vi "Get Hardware ID.vi"() -> ()   [LabVIEW 2012]
panel:
  out "stop":bool
  out "Action":string
  out "p 8":bool
  out "p 7":bool
  out "p 6":bool
  out "p 5":bool
  out "p 4":bool
  out "p 3":bool
  out "p 2":bool
  out "p 1":bool
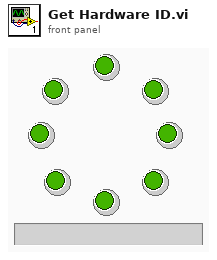
[diagram p1: front panel]
types:
  T1 = enum16{"open", "replace", "create", "open or create", "replace or create", "replace or create with confirmation"}
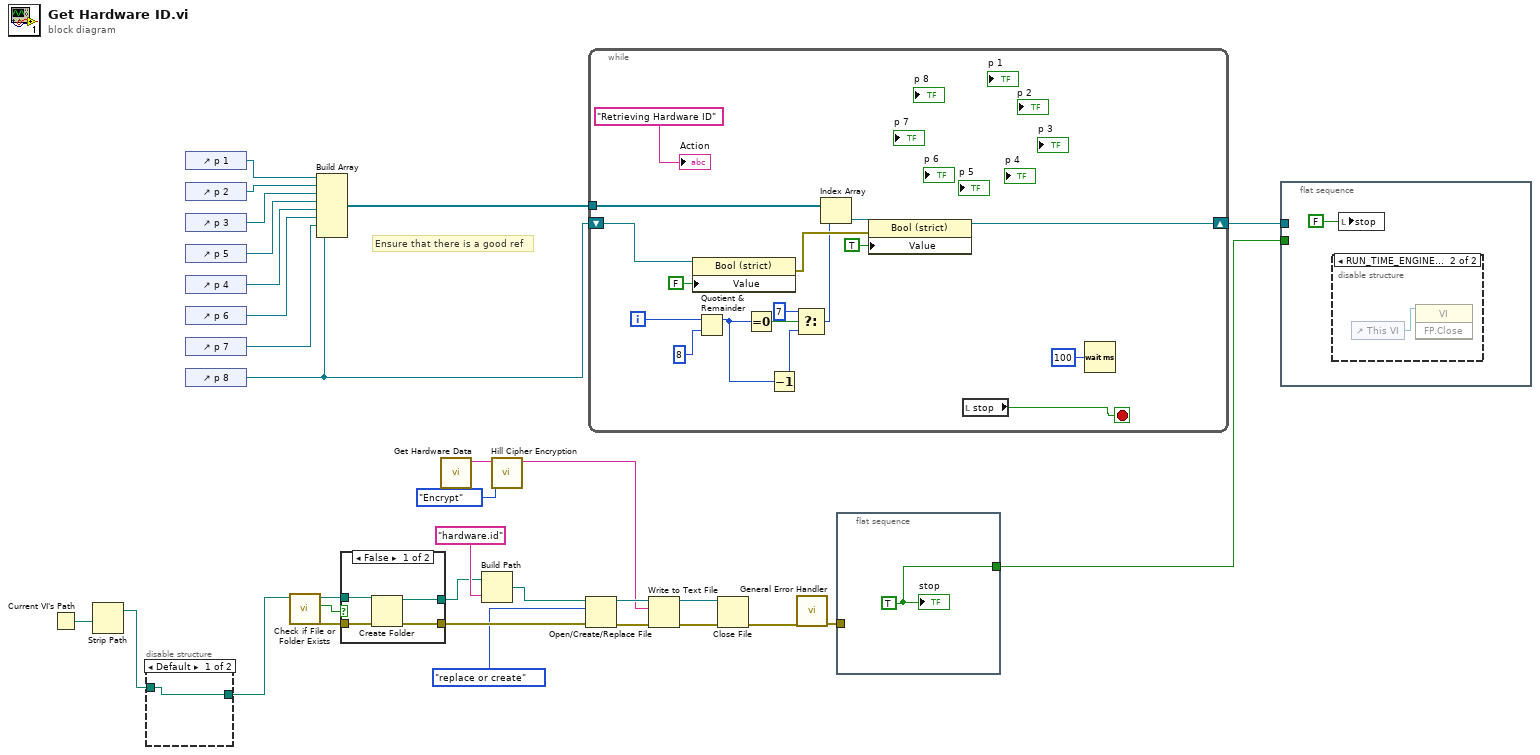
[diagram p0: block diagram]
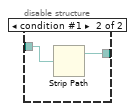
[diagram p2: hidden frame]
diagram:
  # "Ensure that there is a good ref"
  n1 = Current VI's Path() -> (path=w4:path)
  n2 = Strip Path(path=w4) -> (stripped path=w3:path)  [unwired: 1 out]
  n3 = disable-structure shown="Default" {
    disable-tunnel: w3 -> [w32 w34]
    disable-tunnel: [w32 w33] -> w2
    frame condition #0 (active) {
    }
    frame condition #1 {
      n4 = Strip Path(path=w34) -> (stripped path=w33:path)  [unwired: 1 out]
    }
  }
  n5 = control-ref of="p 1"() -> (w8:refnum<vi>)
  n6 = control-ref of="p 2"() -> (w16:refnum<vi>)
  n7 = control-ref of="p 3"() -> (w15:refnum<vi>)
  n8 = control-ref of="p 5"() -> (w14:refnum<vi>)
  n9 = control-ref of="p 4"() -> (w13:refnum<vi>)
  n10 = control-ref of="p 6"() -> (w12:refnum<vi>)
  n11 = control-ref of="p 7"() -> (w11:refnum<vi>)
  n12 = control-ref of="p 8"() -> (w5:refnum<vi>)
  n13 = call <vilib>:"Check if File or Folder Exists.vi"("path"=w2) -> ("error out"=w26:errorcluster, "file or folder exists?"=w24:bool, "dup path"=w25:path)  [unwired: 8 in]
  n14 = Build Array(w8, w16, w15, w14, w13, w12, w11, w5) -> (w10:refnum<vi>[])
  n15 = case shown="False" w24 {
    tunnel: w25 -> [w38 w40]
    tunnel: w26 -> [w37 w39]
    tunnel: [w36 w40] -> w29
    tunnel: [w35 w39] -> w27
    frame False {
      n16 = Create Folder(path (use dialog)=w38, error in=w37) -> (created path=w36:path, error out=w35:errorcluster)  [unwired: 1 in, 1 out]
    }
    frame True {
    }
  }
  n17 = call "Get Hardware Data.vi"() -> ("Fingerprint"=w31:string)  [unwired: 11 in]
  n18 = Build Path(base path=w29, name or relative path="hardware.id") -> (appended path=w28:path)
  n19 = call <userlib>:"Hill Cipher Encryption.vi"("Operation"=enum16{"Encrypt", "Decrypt", "Decrypt from Hex"}."Encrypt", "Input String"=w31) -> ("Output String"=w21:string)  [unwired: 7 in, 2 out]
  n20 = Open/Create/Replace File(file path (use dialog)=w28, error in=w27, operation (0:open)=T1."replace or create") -> (refnum out=w22:refnum<file>, error out=w18:errorcluster)  [unwired: 3 in, 1 out]
  n21 = while {
    tunnel: w10 -> [w53]
    shift-right: [w50] -> w7
    shift-left: w5 -> [w48]
    i -> [w55]
    stop <- w57 stop-if-true
    n22 = property class="Bool (strict)"(reference=w48, "Value"=FALSE) -> (error out=w47:errorcluster)  [unwired: 1 in, 1 out]
    n23 = Quotient & Remainder(x=w55, y=8) -> (x-y*floor(x/y)=w46:i32)  [unwired: 1 out]
    n24 = Equal To 0?(x=w46) -> (x = 0?=w45:bool)
    n25 = Decrement(x=w46) -> (x-1=w44:i32)
    n26 = Select(t=7, s=w45, f=w44) -> (s? t:f=w42:i32)
    n27 = Index Array(array=w53, index=w42) -> (element=w52:refnum<vi>)
    n28 = property class="Bool (strict)"(reference=w52, error in=w47, "Value"=TRUE) -> (reference out=w50:refnum<vi>)  [unwired: 1 out]
    n29 = local read "stop"() -> (w57:bool)
    n30 = Wait (ms)(milliseconds to wait=u32 100) -> ()  [unwired: 1 out]
    "Action" <- "Retrieving Hardware ID" ("Action")
  }
  n31 = Write to Text File(file (use dialog)=w22, text=w21, error in=w18) -> (refnum out=w20:refnum<file>, error out=w19:errorcluster)  [unwired: 1 in, 1 out]
  n32 = Close File(refnum=w20, error in=w19) -> (error out=w17:errorcluster)  [unwired: 1 out]
  n33 = call <vilib>:"General Error Handler.vi"("error in (no error)"=w17) -> ("error out"=w9:errorcluster)  [unwired: 10 in, 4 out]
  n34 = flat-sequence {
    tunnel: [w58] -> w6
    tunnel: w9 -> [_]
    frame #0 {
      w58 = TRUE
      "stop" <- w58
    }
  }
  n35 = flat-sequence {
    tunnel: w7 -> [_]
    tunnel: w6 -> [_]
    frame #0 {
      n36 = disable-structure shown="RUN_TIME_ENGINE==True" {
        frame condition #0 (active) {
        }
        frame condition #1 {
          n37 = control-ref of="This VI"() -> (w60:refnum<vi>)
          n38 = invoke class="VI" method="FP.Close"(reference=w60) -> ()  [unwired: 2 in, 3 out]
        }
      }
      n39 = local write "stop"(FALSE ("stop")) -> ()
    }
  }
